vi "temalabor_pre.vi"() -> ()   [LabVIEW 2013]
panel:
  out "Intensity Graph":i16[][](graph)
  in  "Kepfrissites(Hz)":dbl
  out "Sorelterites(Hz)":dbl
  out "Oszolopelterites(Hz)":dbl
  out "Sorelterites":dynamicdata(graph)
  out "Oszolopelterites":dynamicdata(graph)
  in  "stop":bool
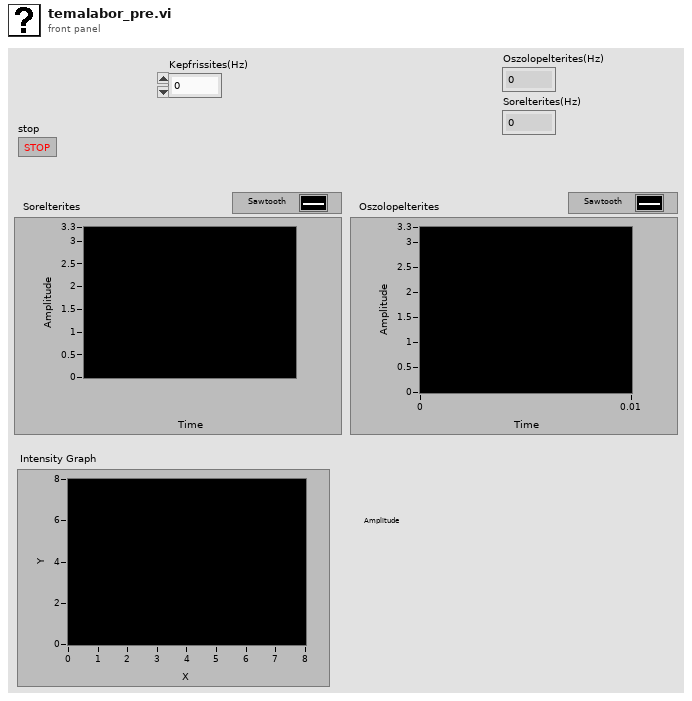
[diagram p1: front panel]
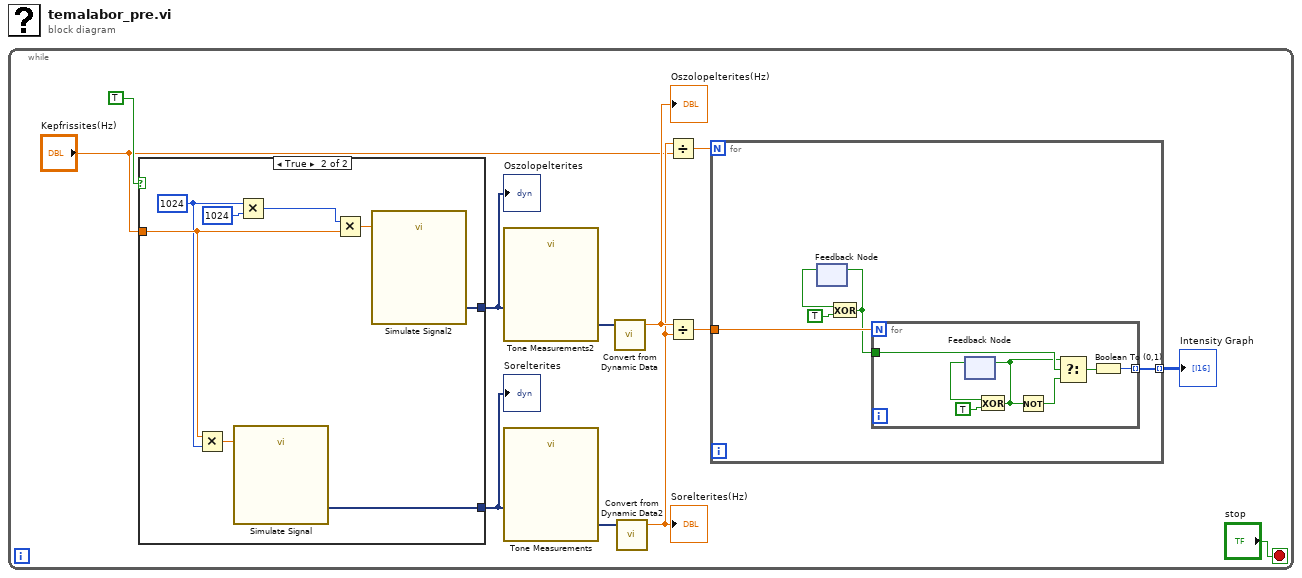
[diagram p0: block diagram]
diagram:
  n1 = while {
    stop <- "stop" stop-if-true
    n2 = case shown="True" TRUE {
      tunnel: [_ w32] -> w11
      tunnel: [_ w31] -> w10
      tunnel: "Kepfrissites(Hz)" -> [_ w26]
      frame False {
      }
      frame True {
        w25 = 1024
        n3 = Multiply(x=w26, y=w25) -> (x*y=w30:dbl)
        n4 = call "Simulate Signal"("Frequency"=w30) -> ("Sawtooth"=w32:dynamicdata)  [unwired: 13 in, 1 out]
        n5 = Multiply(x=w25, y=1024) -> (x*y=w27:i32)
        n6 = Multiply(x=w27, y=w26) -> (x*y=w29:dbl)
        n7 = call "Simulate Signal2"("Frequency"=w29) -> ("Sawtooth"=w31:dynamicdata)  [unwired: 13 in, 1 out]
      }
    }
    "Oszolopelterites" <- w10
    "Sorelterites" <- w11
    n8 = call "Tone Measurements2"("Signals"=w10) -> ("Frequency"=w8:dynamicdata)  [unwired: 9 in, 1 out]
    n9 = call "Tone Measurements"("Signals"=w11) -> ("Frequency"=w9:dynamicdata)  [unwired: 9 in, 1 out]
    n10 = call "Convert from Dynamic Data"("Dynamic Data Type"=w8) -> ("Scalar"=w6:dbl)  [unwired: 3 in]
    "Oszolopelterites(Hz)" <- w6
    n11 = call "Convert from Dynamic Data2"("Dynamic Data Type"=w9) -> ("Scalar"=w5:dbl)  [unwired: 3 in]
    "Sorelterites(Hz)" <- w5
    n12 = Divide(x=w5, y="Kepfrissites(Hz)") -> (x/y=w2:dbl)
    n13 = Divide(x=w6, y=w5) -> (x/y=w3:dbl)
    n14 = for {
      N: w2 -> [_]
      tunnel: w3 -> [w17]
      tunnel: [w16] -> w1 mode=indexing
      n15 = feedback #1() -> (w15:bool)  [unwired: 1 in]
      n16 = Exclusive Or(1:TRUE ("y"), 2:w15) -> (0:w13:bool)
      n17 = feedback-in #1(w13) -> ()
      n18 = for {
        N: w17 -> [_]
        tunnel: [w24] -> w16 mode=indexing
        tunnel: w13 -> [w21]
        n19 = feedback #2() -> (w22:bool)  [unwired: 1 in]
        n20 = Exclusive Or(1:TRUE ("y"), 2:w22) -> (0:w18:bool)
        n21 = feedback-in #2(w18) -> ()
        n22 = Not(x=w18) -> (.not. x?=w20:bool)
        n23 = Select(t=w18, s=w21, f=w20) -> (s? t:f=w19:bool)
        n24 = Boolean To (0,1)(Boolean=w19) -> (0, 1=w24:i16)
      }
    }
    "Intensity Graph" <- w1
  }
